vi "avg_trajectory.vi"() -> ()   [LabVIEW 2017]
uses:
  <vilib>/Utility/file.llb/Read Delimited Spreadsheet (DBL).vi
panel:
  out "Graph":cluster{"Locations":dbl[], "Amplitudes":dbl[]}[](graph)
  in  "Select File \nto Average":path=path "" caption="start path"
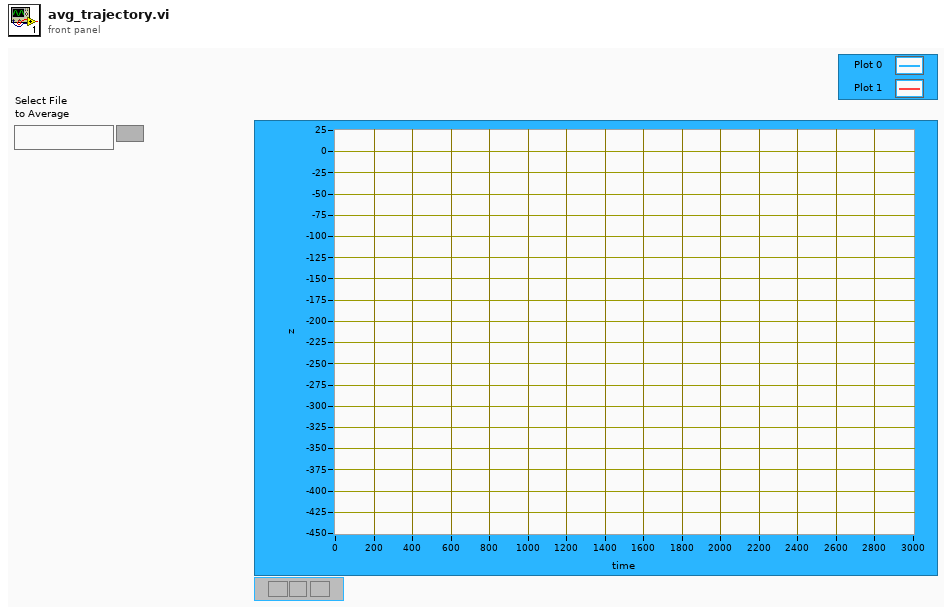
[diagram p1: front panel]
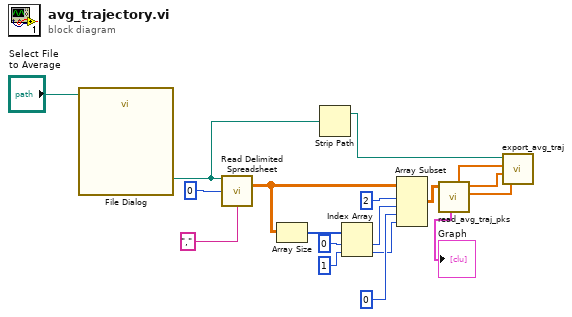
[diagram p0: block diagram]
diagram:
  n1 = call "File Dialog"("start path"="Select File \nto Average") -> ("selected path"=w1:path)  [unwired: 11 in, 3 out]
  n2 = call-poly <vilib>:"Read Delimited Spreadsheet.vi"("file path (dialog if empty)"=w1, "start of read offset (chars.:0)"=0, "delimiter (\\t)"="," ("delimiter (\\t)")) -> ("all rows"=w14:dbl[][])  [unwired: 7 in, 5 out]
  n3 = Array Size(array=w14) -> (size(s)=w13:i32[])
  n4 = Strip Path(path=w1) -> (stripped path=w2:path)  [unwired: 1 out]
  n5 = Index Array(array=w13, index #1=0 ("index"), index #2=1 ("index")) -> (element #1=w11:i32, element #2=w8:i32)
  n6 = Array Subset(array=w14, index (row)=2 ("index"), length (row)=w11, index (col)=0 ("index"), length (col)=w8) -> (w7:dbl[][])
  n7 = call "read_avg_traj_pks.vi"("all rows"=w7) -> ("Graph"=→"Graph":cluster{"Locations":dbl[], "Amplitudes":dbl[]}[], "avg_trajx"=w5:dbl[], "avg_trajy"=w4:dbl[], "avg_trajz"=w3:dbl[])  [unwired: 3 in, 3 out]
  n8 = call "export_avg_traj.vi"("BoundaryZpelv"=w3, "BoundaryYpelv"=w4, "BoundaryXpelv"=w5, "Host folder"=w2) -> ()  [unwired: 1 in]
